vi "Waveform Graph data.vi"(7 "Read N Buffer":string, 8 "Sampling Period":dbl, 9 "Horizontal Position":dbl, 10 "Vertical Scale":dbl, 11 "N Length / 2":dbl) -> (1 "Waveform Start Time":dbl, 2 "Total Waveform Length":i32, 3 "Waveform Graph":cluster{dbl, "Sampling Period":dbl, dbl[]}(graph))   [LabVIEW 2009, in "DSO1K.lvlib"]
doc: "This waveform graph shows the data acquired from the channel."
uses:
  <instrlib>/DSO1K/DSO1K.lvlib
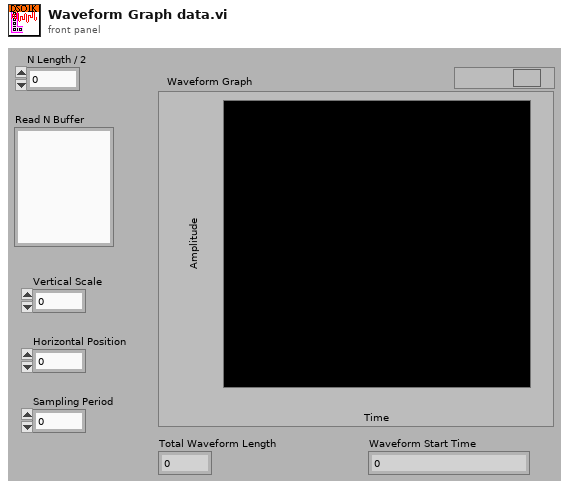
[diagram p1: front panel]
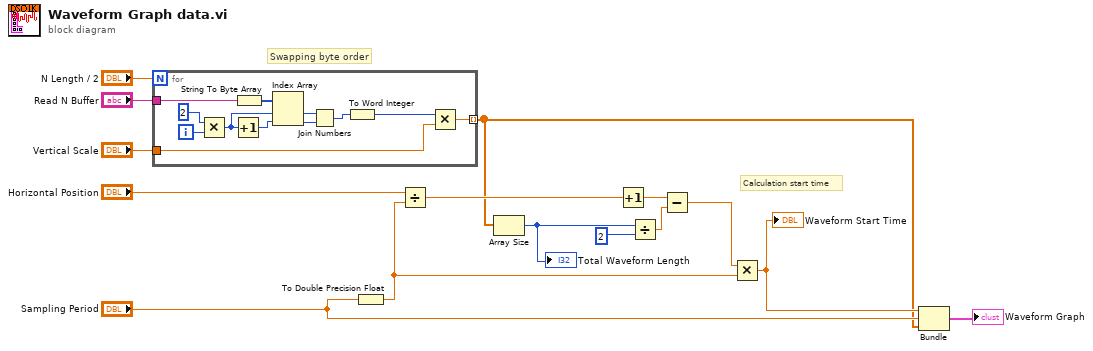
[diagram p0: block diagram]
diagram:
  # "Calculation start time"
  # "Swapping byte order"
  n1 = for {
    N: "N Length / 2" -> [_]
    tunnel: [w21] -> w1 mode=indexing
    tunnel: "Vertical Scale" -> [w20]
    tunnel: "Read N Buffer" -> [w19]
    i -> [w23]
    n2 = Multiply(x=2 ("y"), y=w23) -> (x*y=w27:i32)
    n3 = Increment(x=w27) -> (x+1=w22:i32)
    n4 = String To Byte Array(string=w19) -> (unsigned byte array=w26:u8[])
    n5 = Index Array(array=w26, index #1=w27, index #2=w22) -> (element #1=w18:u8, element #2=w17:u8)
    n6 = Join Numbers(hi=w18, lo=w17) -> ((hi.lo)=w25:u16)
    n7 = To Word Integer(number=w25) -> (16bit integer=w16:i16)
    n8 = Multiply(x=w16, y=w20) -> (x*y=w21:dbl)
  }
  n9 = To Double Precision Float(number="Sampling Period") -> (double precision float=w7:dbl)
  n10 = Divide(x="Horizontal Position", y=w7) -> (x/y=w12:dbl)
  n11 = Array Size(array=w1) -> (size(s)=w6:i32)
  "Total Waveform Length" <- w6
  n12 = Increment(x=w12) -> (x+1=w11:dbl)
  n13 = Divide(x=w6, y=2) -> (x/y=w9:dbl)
  n14 = Subtract(x=w11, y=w9) -> (x-y=w8:dbl)
  n15 = Multiply(x=w8, y=w7) -> (x*y=w5:dbl)
  "Waveform Start Time" <- w5
  n16 = Bundle(w5, "Sampling Period"="Sampling Period", w1) -> (→"Waveform Graph":cluster{dbl, "Sampling Period":dbl, dbl[]})  [unwired: 1 in]
